vi "InTake GetMS.vi"(1 "InTake Global Data In":T1) -> (0 "InTake Global Data Out":T1)   [LabVIEW 2013]
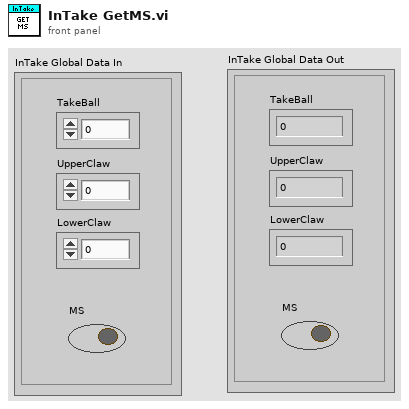
[diagram p1: front panel]
types:
  T1 = cluster{"TakeBall":dbl, "UpperClaw":dbl, "LowerClaw":dbl, "MS":bool}
  T2 = typedef "WPI_DigitalInputDevRef.ctl" = cluster{"DevStatus":errorcluster, "DIO Channel":T3, "Digital Module":T4}
  T3 = typedef "FPGA_DIOChannel.ctl" = enum8{"DIO 1", "DIO 2", "DIO 3", "DIO 4", "DIO 5", "DIO 6", "DIO 7", "DIO 8", "DIO 9", "DIO 10", "DIO 11", "DIO 12", "DIO 13", "DIO 14", "Invalid"}
  T4 = typedef "FPGA_TypedefDigitalModule.ctl" = enum16{"Digital Module 1", "Digital Module 2"}
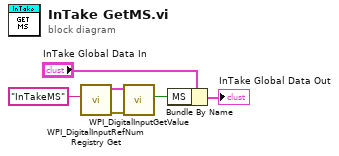
[diagram p0: block diagram]
diagram:
  n1 = call <vilib>:"WPI_DigitalInputRefNum Registry Get.vi"("refnum name"="InTakeMS") -> ("error out"=w3:errorcluster, "DigitalInputDevRef"=w4:T2)  [unwired: 9 in]
  n2 = call <vilib>:"WPI_DigitalInputGetValue.vi"("error in (no error)"=w3, "DigitalInputDevRef"=w4) -> ("Value"=w1:bool)  [unwired: 7 in, 2 out]
  n3 = Bundle By Name(cluster="InTake Global Data In", "MS"=w1) -> (→"InTake Global Data Out":T1)
